vi "Analyze Data.vi"(8 "error in":errorcluster, 11 "PAS in":refnum<class "PAS.lvclass">) -> (0 "error out":errorcluster, 3 "PAS out":refnum<class "PAS.lvclass">)   [LabVIEW 2016, in "PAS Library.lvlib" / "PAS.lvclass"]
doc: "This is the core routine for PAS microphone data analysis. Here, the microphone data is retrieved from each of the cells. In both cases, the time domain signal will be transformed to the frequency domain. If the speaker is on (<B>Spk Pos</B> == TRUE), then the frequency domain signal will be squared to obtain the power and a Lorentzian will be fit to the data to retrieve the resonant characteristics of the cell. If the speaker is off (<B>Spk Pos</B> == FALSE), then the amplitude will be used to calculate the integrated area of the signal. In every case, the implementation has the ability to decimate the data for transmission of the waveforms over a network line."
uses:
  PAS.lvclass
  G:/sw_repo/For Builds/Reusable/Instrument/Instrument.lvclass
  Data/Main/PAS Data.lvclass
  G:/sw_repo/For Builds/Reusable/Data/Data.lvclass
  PAS.lvclass/PAS.ctl
  Instrument/Instrument.lvclass/Instrument.ctl
  Cell/PAS Cell.lvclass/PAS Cell.ctl
  Cell/Read Mod Freq.vi
  Cell/Read filter.vi
  Cell/Read speaker.vi
  Read Chirp.vi
  Instrument/Read Data.vi
  Instrument/Write Data.vi
  Read Cells.vi
  Data/Main/Read CellData.vi
  Cell/Read extParams.vi
  Write Cells.vi
  Data/Data.lvclass
  Cell/PAS Cell.lvclass
  Data/Cell/PAS Cell Data.lvclass
  Instrument/Instrument.lvclass
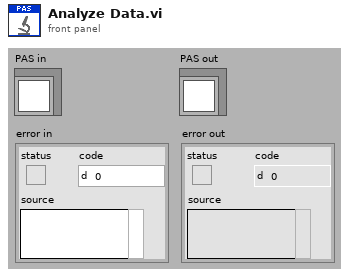
[diagram p1: front panel]
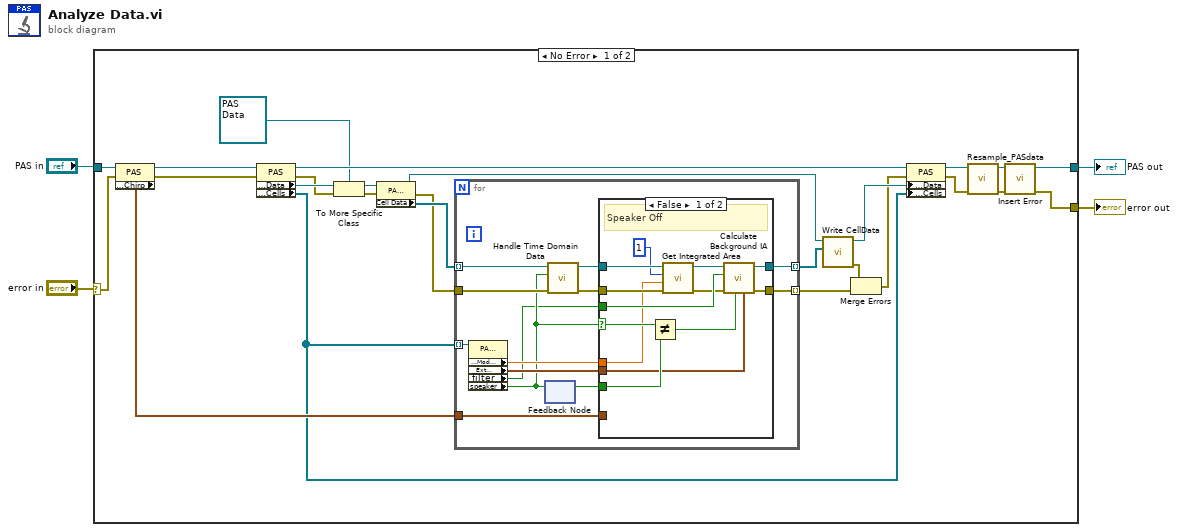
[diagram p0: block diagram]
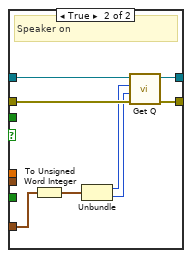
[diagram p2: hidden frame]
diagram:
  n1 = case shown="No Error" "error in" {
    selector: "error in" -> [w25 w66]
    tunnel: [w29 w66] -> w1
    tunnel: [w30 w65] -> w2
    tunnel: "PAS in" -> [w28 w65]
    frame No Error {
      n2 = property class="PAS"(reference=w28, error in=w25) -> (reference out=w27:refnum<class "PAS.lvclass">, error out=w26:errorcluster, "Data Access:Chirp"=w24:cluster{"f_center":dbl, "bandwidth":dbl})
      n3 = property class="PAS"(reference=w27, error in=w26) -> (reference out=w9:refnum<class "PAS.lvclass">, error out=w7:errorcluster, "Accessors:Data"=w11:refnum<class "Data.lvclass">, "Data Access:Cells"=w8:refnum<class "PAS Cell.lvclass">[])
      n4 = To More Specific Class(target class=refnum<class "PAS Data.lvclass"> refnum ("reference"), reference=w11, error in=w7) -> (specific class reference=w13:refnum<class "PAS Data.lvclass">, error out=w12:errorcluster)
      n5 = property class="PAS Data"(reference=w13, error in=w12) -> (reference out=w15:refnum<class "PAS Data.lvclass">, error out=w14:errorcluster, "Cell Data"=w16:refnum<class "PAS Cell Data.lvclass">[])
      n6 = for {
        tunnel: w16 -> [w41] mode=indexing
        tunnel: [w34] -> w19 mode=indexing
        tunnel: [w35] -> w18 mode=indexing
        tunnel: w14 -> [w38]
        tunnel: w8 -> [w43] mode=indexing
        tunnel: w24 -> [w42]
        n7 = property class="PAS Cell"(reference=w43) -> ("Accessors:Mod Freq"=w36:sgl, "Ext Params"=w37:cluster{"slope":sgl, "zero":sgl}, "filter"=w31:bool, "speaker"=w32:bool)  [unwired: 1 in, 2 out]
        n8 = feedback #1() -> (w33:bool)  [unwired: 1 in]
        n9 = feedback-in #1(w32) -> ()
        n10 = call "Handle Time Domain Data.vi"("error in"=w38, "Spkeaker On?"=w32, "Cell Data in"=w41) -> ("error out"=w39:errorcluster, "Cell Data out"=w40:refnum<class "PAS Cell Data.lvclass">)  [unwired: 7 in]
        n11 = case shown="False" w32 {
          selector: w32 -> [w53 _]
          tunnel: w40 -> [w52 w62]
          tunnel: w39 -> [w48 w61]
          tunnel: [w55 w64] -> w35
          tunnel: [w56 w63] -> w34
          tunnel: w37 -> [w45 _]
          tunnel: w42 -> [_ w58]
          tunnel: w31 -> [w54 _]
          tunnel: w33 -> [w47 _]
          tunnel: w36 -> [w46 _]
          frame False {
            # "Speaker Off"
            n12 = Not Equal?(x=w53, y=w47) -> (x != y?=w44:bool)
            n13 = call "Get Integrated Area.vi"("error in"=w48, "fmod"=w46, "p"=1 ("Integrated Area"), "PAS Cell Data in"=w52) -> ("error out"=w50:errorcluster, "PAS Cell Data out"=w51:refnum<class "PAS Cell Data.lvclass">)  [unwired: 6 in]
            n14 = call "Calculate Background IA.vi"("Fit Params"=w45, "Sw From Spk"=w44, "error in"=w50, "Filter"=w54, "Cell Data in"=w51) -> ("error out"=w55:errorcluster, "Cell Data out"=w56:refnum<class "PAS Cell Data.lvclass">)  [unwired: 5 in]
          }
          frame True {
            # "Speaker on"
            n15 = To Unsigned Word Integer(number=w58) -> (unsigned 16bit integer=w57:cluster{"f_center":u16, "bandwidth":u16})
            n16 = Unbundle(w57) -> ("f_center"=w60:u16, "bandwidth"=w59:u16)
            n17 = call "Get Q.vi"("error in"=w61, "Bandwidth"=w59, "f_center"=w60, "PAS Cell Data in"=w62) -> ("error out"=w64:errorcluster, "PAS Cell Data out"=w63:refnum<class "PAS Cell Data.lvclass">)  [unwired: 6 in]
          }
        }
      }
      n18 = call "Write CellData.vi"("CellData"=w19, "PAS Data in"=w15) -> ("error out"=w17:errorcluster, "PAS Data out"=w10:refnum<class "PAS Data.lvclass">)  [unwired: 8 in]
      n19 = Merge Errors(w17, w18) -> (w6:errorcluster)
      n20 = property class="PAS"(reference=w9, error in=w6, "Accessors:Data"=w10, "Data Access:Cells"=w8) -> (reference out=w23:refnum<class "PAS.lvclass">, error out=w21:errorcluster)
      n21 = call "Resample_PASdata.vi"("error in"=w21, "PAS in"=w23) -> ("error out"=w20:errorcluster, "PAS out"=w22:refnum<class "PAS.lvclass">)  [unwired: 8 in]
      n22 = call "Insert Error.vi"("error in"=w20, "Instrument in"=w22) -> ("error out"=w29:errorcluster, "Instrument out"=w30:refnum<class "PAS.lvclass">)  [unwired: 7 in, 1 out]
    }
    frame Error {
    }
  }
  "error out" <- w1
  "PAS out" <- w2
